vi "Create_Deadband.vi"(2 "Output Lower Limit":dbl, 3 "Input":dbl, 4 "Output Upper Limit":dbl=1.0 format="%#_13g") -> (0 "Output":dbl, 1 "Not Zero?":bool)   [LabVIEW 2018]
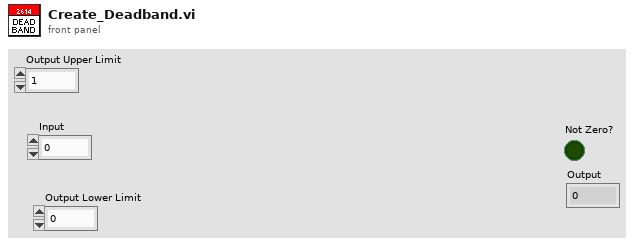
[diagram p1: front panel]
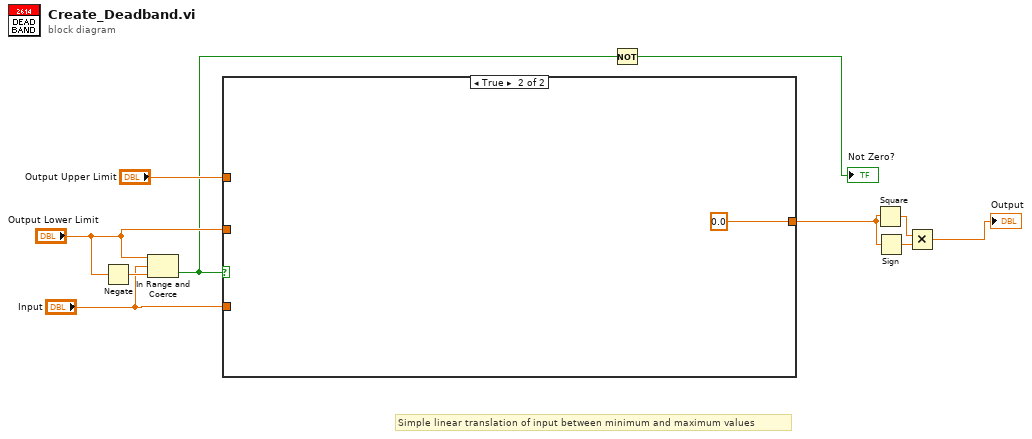
[diagram p0: block diagram]
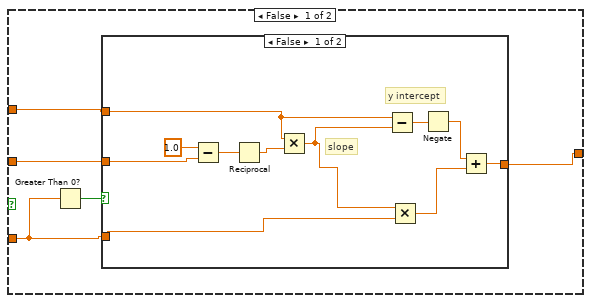
[diagram p2: hidden frame]
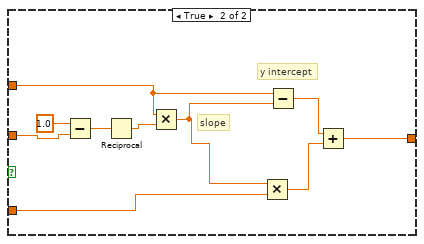
[diagram p3: hidden frame]
diagram:
  # "Simple linear translation of input between minimum and maximum values"
  n1 = Negate(x="Output Lower Limit") -> (-x=w10:dbl)
  n2 = In Range and Coerce(upper limit="Output Lower Limit", x="Input", lower limit=w10) -> (In Range?=w6:bool)  [unwired: 1 out]
  n3 = case shown="True" w6 {
    tunnel: "Output Lower Limit" -> [w14 _]
    tunnel: "Input" -> [w11 _]
    tunnel: [w13 0.0 ("Output")] -> w2
    tunnel: "Output Upper Limit" -> [w15 _]
    frame False {
      n4 = Greater Than 0?(x=w11) -> (x > 0?=w12:bool)
      n5 = case shown="False" w12 {
        tunnel: w15 -> [w21 w33]
        tunnel: w14 -> [w22 w32]
        tunnel: w11 -> [w20 w31]
        tunnel: [w19 w28] -> w13
        frame False {
          # "y intercept"
          # "slope"
          n6 = Subtract(x=1.0, y=w22) -> (x-y=w24:dbl)
          n7 = Reciprocal(x=w24) -> (1/x=w25:dbl)
          n8 = Multiply(x=w21, y=w25) -> (x*y=w16:dbl)
          n9 = Subtract(x=w21, y=w16) -> (x-y=w18:dbl)
          n10 = Multiply(x=w16, y=w20) -> (x*y=w26:dbl)
          n11 = Negate(x=w18) -> (-x=w17:dbl)
          n12 = Add(x=w17, y=w26) -> (x+y=w19:dbl)
        }
        frame True {
          # "y intercept"
          # "slope"
          n13 = Subtract(x=1.0, y=w32) -> (x-y=w35:dbl)
          n14 = Reciprocal(x=w35) -> (1/x=w34:dbl)
          n15 = Multiply(x=w33, y=w34) -> (x*y=w27:dbl)
          n16 = Multiply(x=w27, y=w31) -> (x*y=w30:dbl)
          n17 = Subtract(x=w33, y=w27) -> (x-y=w29:dbl)
          n18 = Add(x=w29, y=w30) -> (x+y=w28:dbl)
        }
      }
    }
    frame True {
    }
  }
  n19 = Not(x=w6) -> (.not. x?=→"Not Zero?":bool)
  n20 = Square(x=w2) -> (x^2=w4:dbl)
  n21 = Sign(1:w2) -> (0:w3:dbl)
  n22 = Multiply(x=w4, y=w3) -> (x*y=→"Output":dbl)
